vi "GrayToRGB-CSV.vi"() -> ()   [LabVIEW 2019]
uses:
  Control 1.ctl
  Gray_To_RGB DLL Project/Project Library For VI/Gray_to_RGB.dll
panel:
  in  "Available Colormaps":T1
  in  "CSV File Path":path
  out "RGB Image":T2(plugin-control)
  out "Elapsed Time in C":dbl
  out "Gray Image":T2(plugin-control)
  in  "Gray Image Path":path
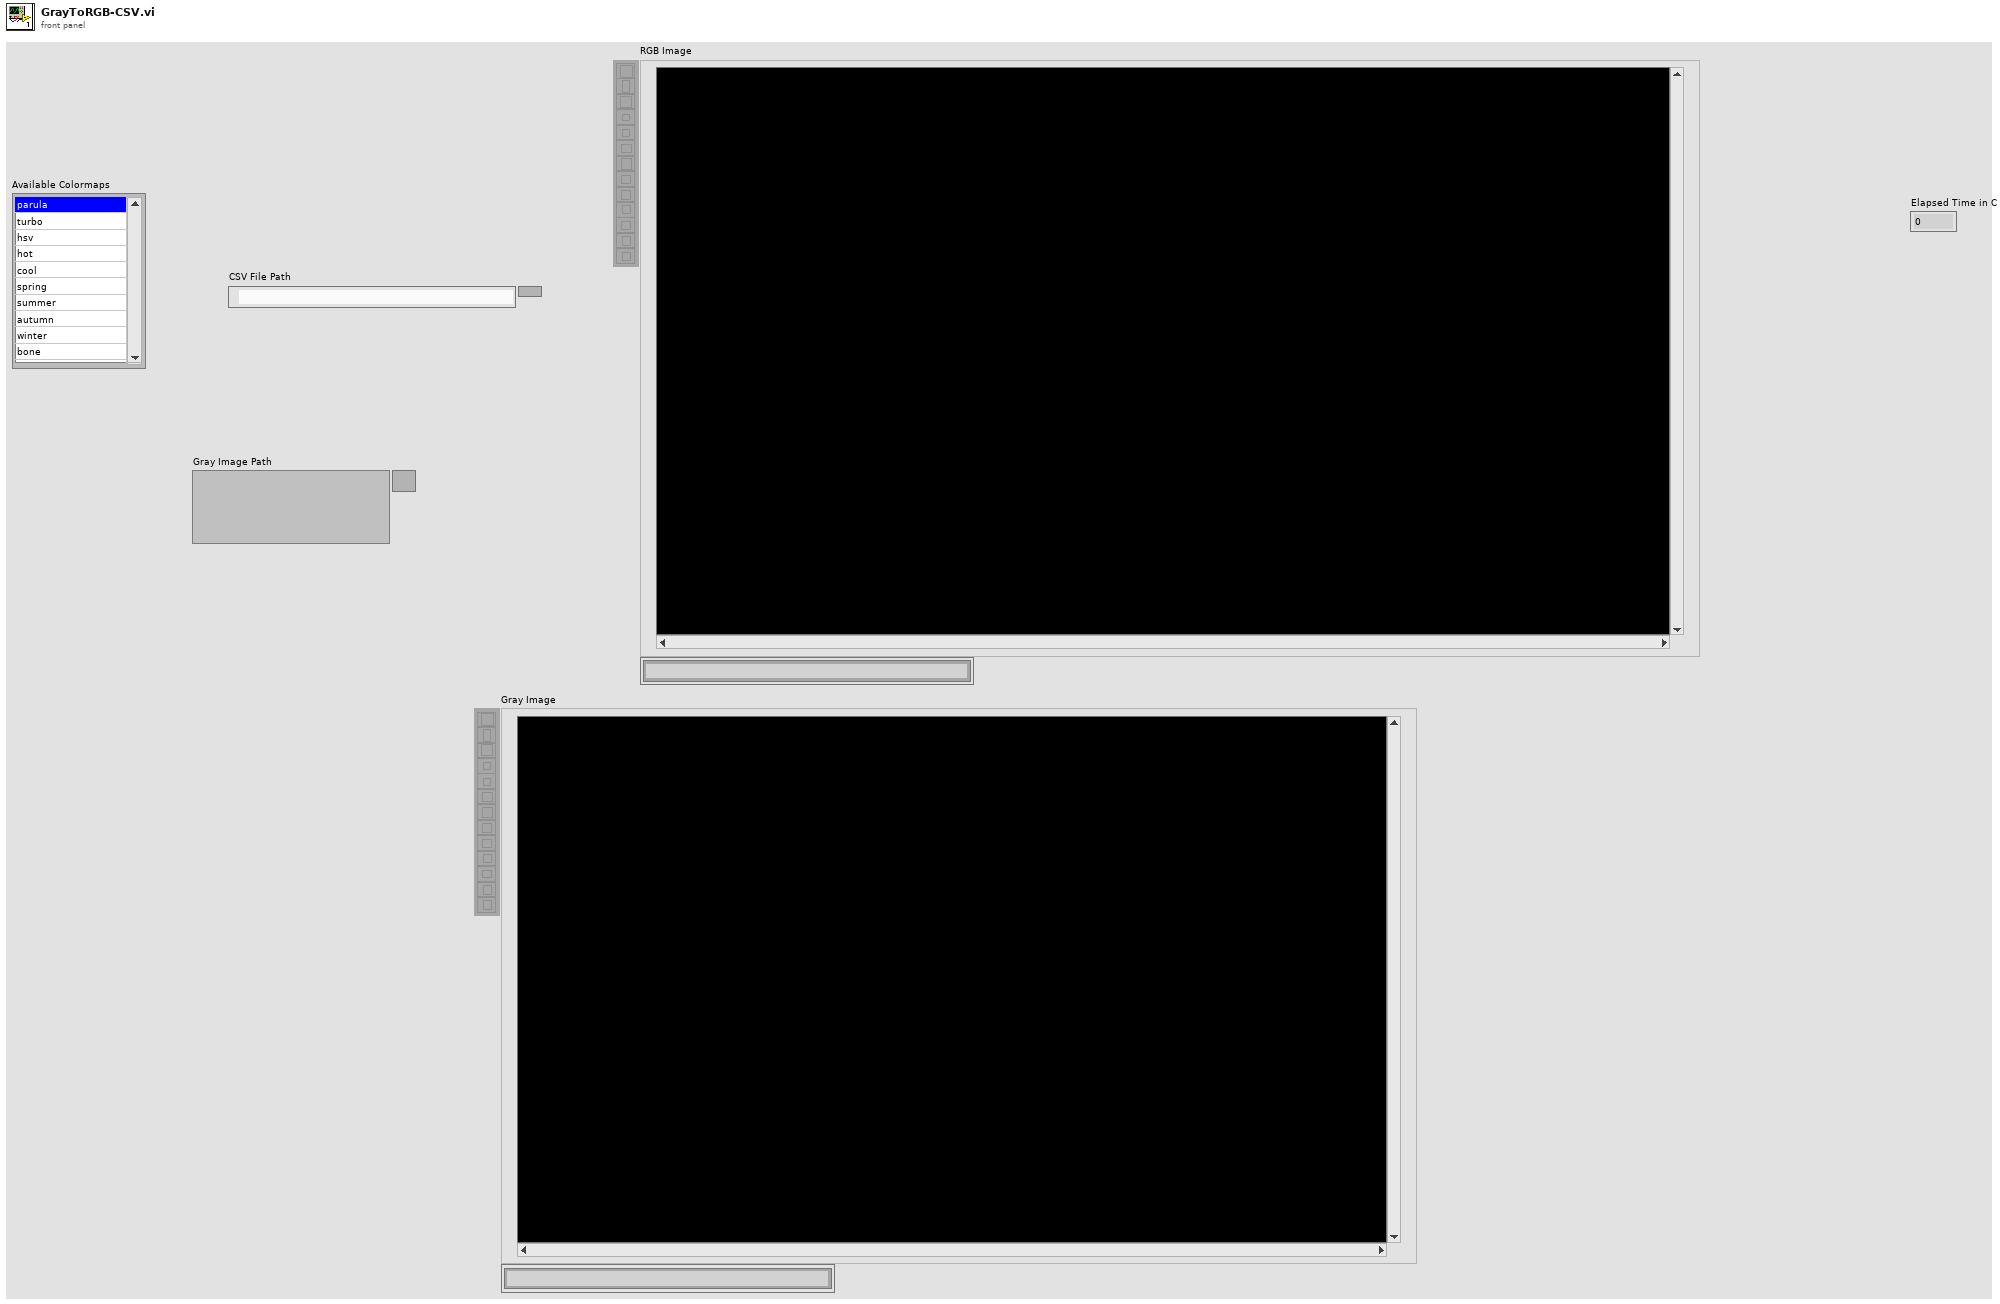
[diagram p1: front panel]
types:
  T1 = typedef "Control 1.ctl" = i32
  T2 = typedef "IMAQ Image.ctl" = refnum<image>
  T3 = enum32{"Map Pixel Pointer", "Unmap Pixel Pointer", "Get Pixels Infos"}
  T4 = typedef "Image Type" = u32
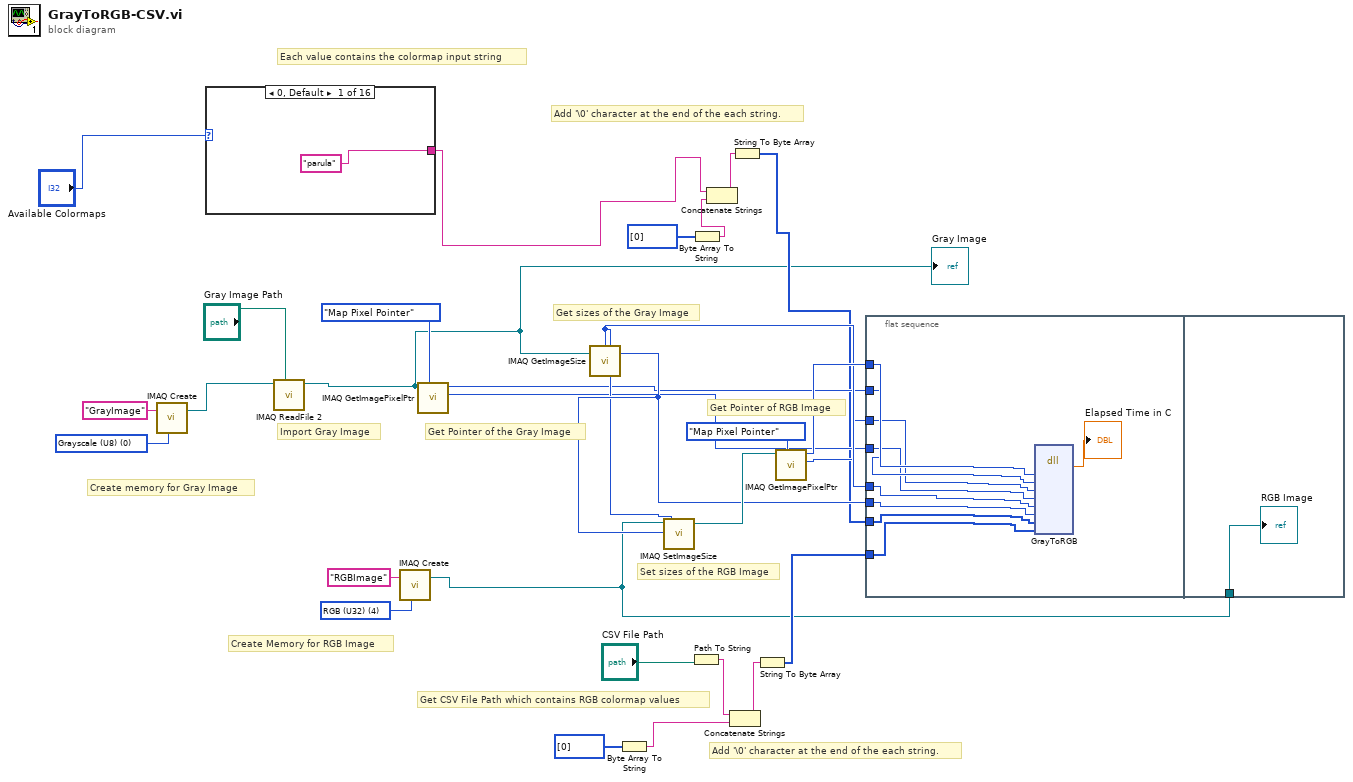
[diagram p0: block diagram]
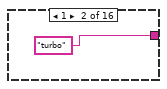
[diagram p2: hidden frame]
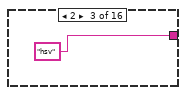
[diagram p3: hidden frame]
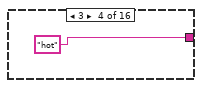
[diagram p4: hidden frame]
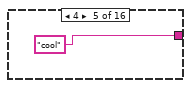
[diagram p5: hidden frame]
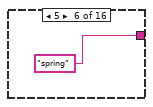
[diagram p6: hidden frame]
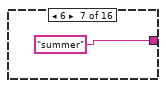
[diagram p7: hidden frame]
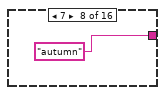
[diagram p8: hidden frame]
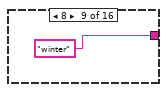
[diagram p9: hidden frame]
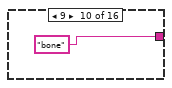
[diagram p10: hidden frame]
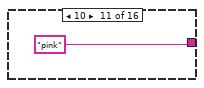
[diagram p11: hidden frame]
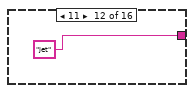
[diagram p12: hidden frame]
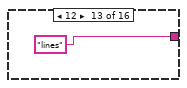
[diagram p13: hidden frame]
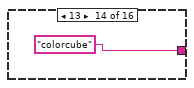
[diagram p14: hidden frame]
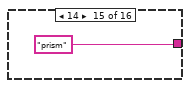
[diagram p15: hidden frame]
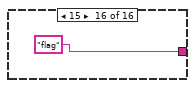
[diagram p16: hidden frame]
diagram:
  w23 = T4 4 items=["Grayscale (U8)", "Grayscale (I16)", "Grayscale (SGL)", "Complex (CSG)", "RGB (U32)", "HSL (U32)", "RGB (U64)", "Grayscale (U16)"] ("Image Type")
  w27 = T4 0 items=["Grayscale (U8)", "Grayscale (I16)", "Grayscale (SGL)", "Complex (CSG)", "RGB (U32)", "HSL (U32)", "RGB (U64)", "Grayscale (U16)"] ("Image Type")
  # "Each value contains the colormap input string"
  # "Get Pointer of RGB Image"
  # "Set sizes of the RGB Image"
  # "Get CSV File Path which contains RGB colormap values"
  # "Create Memory for RGB Image"
  # "Get sizes of the Gray Image"
  # "Get Pointer of the Gray Image"
  # "Import Gray Image"
  # "Create memory for Gray Image"
  # "Add '\\0' character at the end of the each string."
  # "Add '\\0' character at the end of the each string."
  n1 = call "IMAQ Create"("Image Name"="GrayImage", "Image Type"=w27) -> ("New Image"=w26:T2)  [unwired: 3 in, 1 out]
  n2 = case shown="0, Default" "Available Colormaps" {
    tunnel: ["parula" "turbo" "hsv" "hot" "cool" "spring" "summer" "autumn" "winter" "bone" "pink" "jet" "lines" "colorcube" "prism" "flag"] -> w9
    frame 0, Default {
    }
    frame 1 {
    }
    frame 2 {
    }
    frame 3 {
    }
    frame 4 {
    }
    frame 5 {
    }
    frame 6 {
    }
    frame 7 {
    }
    frame 8 {
    }
    frame 9 {
    }
    frame 10 {
    }
    frame 11 {
    }
    frame 12 {
    }
    frame 13 {
    }
    frame 14 {
    }
    frame 15 {
    }
  }
  n3 = call "IMAQ ReadFile 2"("File Path"="Gray Image Path", "Image"=w26) -> ("Image Out"=w1:T2)  [unwired: 5 in, 4 out]
  "Gray Image" <- w1
  n4 = call "IMAQ Create"("Image Name"="RGBImage", "Image Type"=w23) -> ("New Image"=w2:T2)  [unwired: 3 in, 1 out]
  n5 = call "IMAQ GetImagePixelPtr"("Function"=T3."Map Pixel Pointer", "Image"=w1) -> ("LineWidth(Pixels)"=w16:i32, "Pixel Pointer out"=w17:u64)  [unwired: 4 in, 4 out]
  n6 = call "IMAQ GetImageSize"("Image"=w1) -> ("Y Resolution"=w20:i32, "X Resolution"=w18:i32)  [unwired: 3 in, 1 out]
  n7 = Byte Array To String(unsigned byte array=u8[] [0]) -> (string=w4:string)
  n8 = call "IMAQ SetImageSize"("Y Resolution"=w20, "X Resolution"=w18, "Image"=w2) -> ("Image Out"=w22:T2)  [unwired: 2 in, 1 out]
  n9 = Path To String(path="CSV File Path") -> (string=w5:string)
  n10 = Byte Array To String(unsigned byte array=u8[] [0]) -> (string=w8:string)
  n11 = Concatenate Strings(w9, w8) -> (w7:string)
  n12 = Concatenate Strings(w5, w4) -> (w3:string)
  n13 = String To Byte Array(string=w7) -> (unsigned byte array=w14:u8[])
  n14 = String To Byte Array(string=w3) -> (unsigned byte array=w13:u8[])
  n15 = call "IMAQ GetImagePixelPtr"("Function"=T3."Map Pixel Pointer", "Image"=w22) -> ("LineWidth(Pixels)"=w15:i32, "Pixel Pointer out"=w19:u64)  [unwired: 4 in, 4 out]
  n16 = flat-sequence {
    tunnel: w20 -> [w49]
    tunnel: w18 -> [w50]
    tunnel: w19 -> [w54]
    tunnel: w17 -> [w53]
    tunnel: w16 -> [w51]
    tunnel: w15 -> [w52]
    tunnel: w14 -> [w48]
    tunnel: w13 -> [w47]
    tunnel: w2 -> [w55]
    frame #0 {
      n17 = dll-call lib="C:/Users/DELL/Desktop/EE433/EE-433 Project Group1/Gray_To_RGB DLL Project/Project Library For VI/Gray_to_RGB.dll" fn="GrayToRGB"("RGBImage"=w54, "GrayImage"=w53, "LVLineWidthRGB"=w52, "LVLineWidthGray"=w51, "LVWidth"=w50, "LVHeight"=w49, "ColorMap"=w48, "CsvPath"=w47) -> ("return type"=→"Elapsed Time in C":dbl)  [unwired: 11 in, 2 out]
    }
    frame #1 {
      "RGB Image" <- w55
    }
  }
